vi "Get Value as Variant.vi"(8 "error in (no error)":errorcluster, 11 "CVT_String in":refnum<class "CVT_String.lvclass">) -> (0 "error out":errorcluster, 2 "data":variant, 3 "CVT_String out":refnum<class "CVT_String.lvclass">)   [LabVIEW 2024, in "Current Value Table.lvlib" / "CVT_String.lvclass"]
uses:
  CVT_String.lvclass
  CVT_String.lvclass/CVT_String.ctl
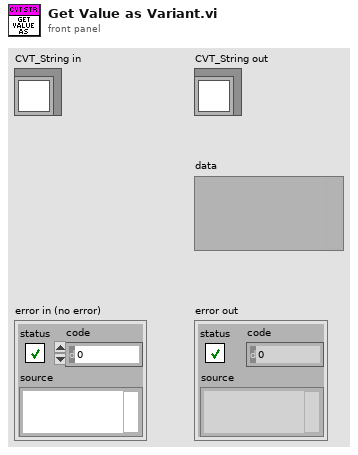
[diagram p1: front panel]
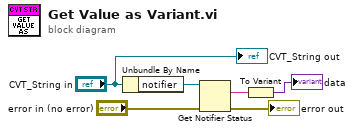
[diagram p0: block diagram]
diagram:
  n1 = Unbundle By Name("CVT_String in") -> ("notifier"=w5:refnum<notifier>)
  n2 = Get Notifier Status(notifier=w5, error in (no error)="error in (no error)") -> (current notification=w3:string, error out=→"error out":errorcluster)  [unwired: 3 out]
  n3 = To Variant(anything=w3) -> (Variant=→"data":variant)
  "CVT_String out" <- "CVT_String in"
